vi "test Write.vi"(11 "Test Case In":refnum<class "Tests Event MessengerM.lvclass">) -> (0 "error out":errorcluster, 3 "Test Case Out":refnum<class "Tests Event MessengerM.lvclass">)   [LabVIEW 2020, in "Tests Event MessengerM.lvclass"]
uses:
  Tests Event MessengerM.lvclass
  C:/Program Files/National Instruments/LabVIEW 2025/vi.lib/Astemes/LUnit/Test Case.lvclass
  <vilib>/Astemes/LUnit/Test Case.lvclass/Test Case.ctl
  <vilib>/Astemes/LUnit/Core/LUnit Test Case/Private/Append Fail Result.vi
  <vilib>/Astemes/LUnit/Core/LUnit Test Case/Private/Append Pass Result.vi
  <vilib>/Astemes/LUnit/Core/LUnit Test Case/Private/Run In UI.vi
  <vilib>/Utility/error.llb/Clear Errors.vi
  source/Instantiate.vi
  source/))Channel.vi
  source/Event MessengerM.lvlib
  <vilib>/Astemes/LUnit/Test Case.lvclass
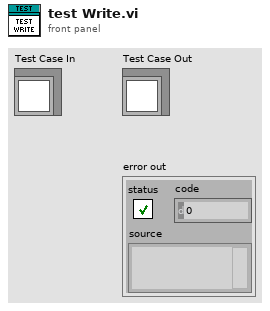
[diagram p1: front panel]
types:
  T1 = typedef "Event MessengerM.lvlib/))Channel.ctl" = refnum<queue>
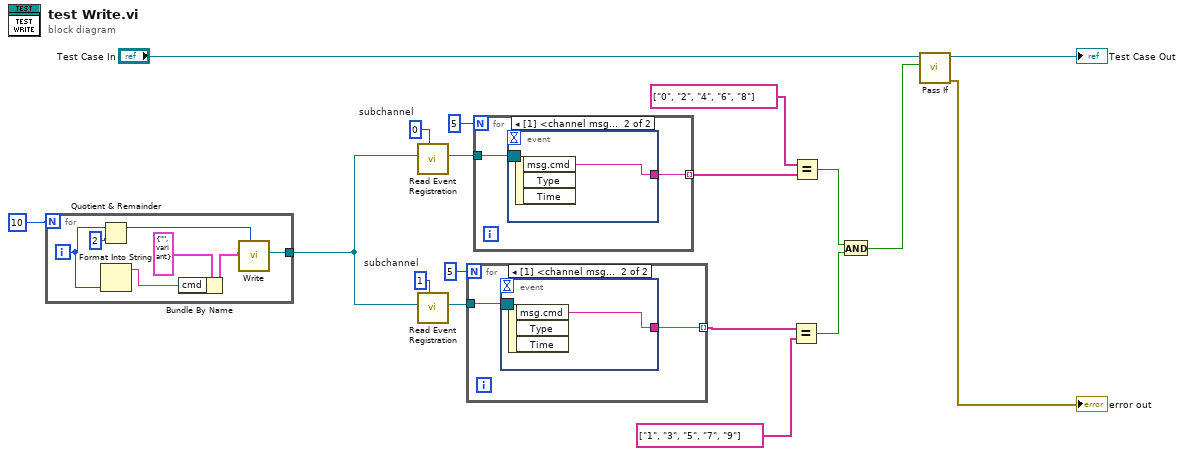
[diagram p0: block diagram]
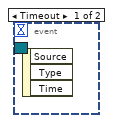
[diagram p2: hidden frame]
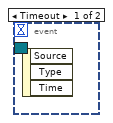
[diagram p3: hidden frame]
diagram:
  w12 = 1  # subchannel
  w14 = 0  # subchannel
  n1 = for {
    N: 10 -> [_]
    tunnel: [w25] -> w13
    i -> [w20]
    n2 = Quotient & Remainder(x=w20, y=2) -> (x-y*floor(x/y)=w23:i32)  [unwired: 1 out]
    n3 = Format Into String(w20) -> (resulting string=w19:string)  [unwired: 3 in, 1 out]
    n4 = Bundle By Name(cluster=cluster{"cmd":string, "data":variant} {"cmd"="", "data"=variant} ("element"), "cmd"=w19) -> (w21:cluster{"cmd":string, "data":variant})
    n5 = call "Write.vi"("subchannel (0)"=w23, "element"=w21) -> ("channel"=w25:T1)  [unwired: 8 in, 1 out]
  }
  n6 = call "Read Event Registration.vi"("subchannel"=w14, "channel"=w13) -> ("event registration refnum"=w11:refnum<event-registration>)  [unwired: 9 in]
  n7 = call "Read Event Registration.vi"("subchannel"=w12, "channel"=w13) -> ("event registration refnum"=w10:refnum<event-registration>)  [unwired: 9 in]
  n8 = for {
    N: 5 -> [_]
    tunnel: w10 -> [w27]
    tunnel: [w26] -> w7 mode=indexing
    n9 = event shown="[1] <channel msg>: User Event" {
      selector: w27 -> [_ _]
      dyn-events: _ -> [_ _]
      timeout: _ -> [_ _]
      tunnel: [_ w28] -> w26
      event Timeout {
        n10 = event-data() -> ()  [unwired: 1 in, 3 out]
      }
      event User Event {
        n11 = event-data() -> ("msg.cmd"=w28:string)  [unwired: 1 in, 2 out]
      }
    }
  }
  n12 = for {
    N: 5 -> [_]
    tunnel: w11 -> [w30]
    tunnel: [w29] -> w4 mode=indexing
    n13 = event shown="[1] <channel msg>: User Event" {
      selector: w30 -> [_ _]
      dyn-events: _ -> [_ _]
      timeout: _ -> [_ _]
      tunnel: [_ w31] -> w29
      event Timeout {
        n14 = event-data() -> ()  [unwired: 1 in, 3 out]
      }
      event User Event {
        n15 = event-data() -> ("msg.cmd"=w31:string)  [unwired: 1 in, 2 out]
      }
    }
  }
  n16 = Equal?(x=w7, y=string[] ["1", "3", "5", "7", "9"] ("Array 2")) -> (x = y?=w5:bool)
  n17 = Equal?(x=string[] ["0", "2", "4", "6", "8"] ("Array"), y=w4) -> (x = y?=w2:bool)
  n18 = And(x=w2, y=w5) -> (x .and. y?=w1:bool)
  n19 = call <vilib>:"Pass If.vi"("Pass?"=w1, "LUnit Test Case In"="Test Case In") -> ("error out"=→"error out":errorcluster, "LUnit Test Case Out"=→"Test Case Out":refnum<class "Tests Event MessengerM.lvclass">)  [unwired: 8 in]
